vi "Scale_FPGA_Output_To_Volts.vi"(7 "Chan#":T8, 10 "FPGA_Data":ext[](array[numeric]), 11 "FP_User":T1={"#NoiseSums"=0, "Max_df"=0, "AvgAvg"=FALSE, "#Avg"=0, "AutoCenter"=FALSE, "Inclin"={"Vmin"=0.0, "Vmax"=0.0, "Angle_min"=0.0, "Angle_max"=0.0, "Offset"=0.0, "Pos_Neg"=FALSE}, "1"={"Cal_"={"Fine"=0.0, "Coarse_"=0.0}, "Beac"={"Fine"=0.0, "Coarse_"=0.0}, "Scale"={"Step4"=0.0, "Step5"=0.0, "Step6"=0.0, "Step7"=0.0}, "Offset"=0.0, "Scale_Noise"=0.0, "Scale_Step1"=0.0, "Scale_In_RT"=0.0, "ScaleMeas"=0.0, "FreqsToRemove"=[], "Width"=[0, 1633], "ScaleMeasEnum"=enum."1", "FilterEnab"=enum."None"}, "2"={"Cal_"={"Fine"=0.0, "Coarse_"=0.0}, "Beac"={"Fine"=0.0, "Coarse_"=0.0}, "Scale"={"Step4"=0.0, "Step5"=0.0, "Step6"=0.0, "Step7"=0.0}, "Offset"=0.0, "Scale_Noise"=0.0, "Scale_Step1"=0.0, "Scale_In_RT"=0.0, "ScaleMeas"=0.0, "FreqsToRemove"=[], "Width"=[0, 1633], "ScaleMeasEnum"=enum."1", "FilterEnab"=enum."None"}, "3"={"Cal_"={"Fine"=0.0, "Coarse_"=0.0}, "Beac"={"Fine"=0.0, "Coarse_"=0.0}, "Scale"={"Step4"=0.0, "Step5"=0.0, "Step6"=0.0, "Step7"=0.0}, "Offset"=0.0, "Scale_Noise"=0.0, "Scale_Step1"=0.0, "Scale_In_RT"=0.0, "ScaleMeas"=0.0, "FreqsToRemove"=[], "Width"=[0, 1633], "ScaleMeasEnum"=enum."1", "FilterEnab"=enum."None"}, "4"={"Cal_"={"Fine"=0.0, "Coarse_"=0.0}, "Beac"={"Fine"=0.0, "Coarse_"=0.0}, "Scale"={"Step4"=0.0, "Step5"=0.0, "Step6"=0.0, "Step7"=0.0}, "Offset"=0.0, "Scale_Noise"=0.0, "Scale_Step1"=0.0, "Scale_In_RT"=0.0, "ScaleMeas"=0.0, "FreqsToRemove"=[], "Width"=[0, 1633], "ScaleMeasEnum"=enum."1", "FilterEnab"=enum."None"}, "Target to Probe"=enum."1", "SNR_Thresh"=0.0, "Paths"={"CfgFile"=path "", "LogFolder"=path "", "LogFile"=path "", "NAS path"=path "", "ThreshFile"=path "", "RedunFolder"=path ""}, "Connex_Location"="", "SimulateFPGA"=FALSE, "Deadband"=0.0} {"Deadband" format="%#.0f"}) -> (2 "VoltsScalar":dbl, 3 "Time Domain Volts":ext[](array[numeric]))   [LabVIEW 2018]
uses:
  Controls/Enums/TargetNumber.ctl
  Controls/Clusts/FrontPanel_UserConfig.ctl
  Controls/Clusts/Inclinometer_User_Cfg.ctl
  Controls/Clusts/FP_UserTargetConfig.ctl
  Controls/Clusts/FreqShift.ctl
  Controls/Clusts/FPGA_Scale.ctl
  Controls/Enums/ScaleMeasure.ctl
  Controls/RadioButtons/FilterEnableRadio.ctl
  Controls/PathsCluster.ctl
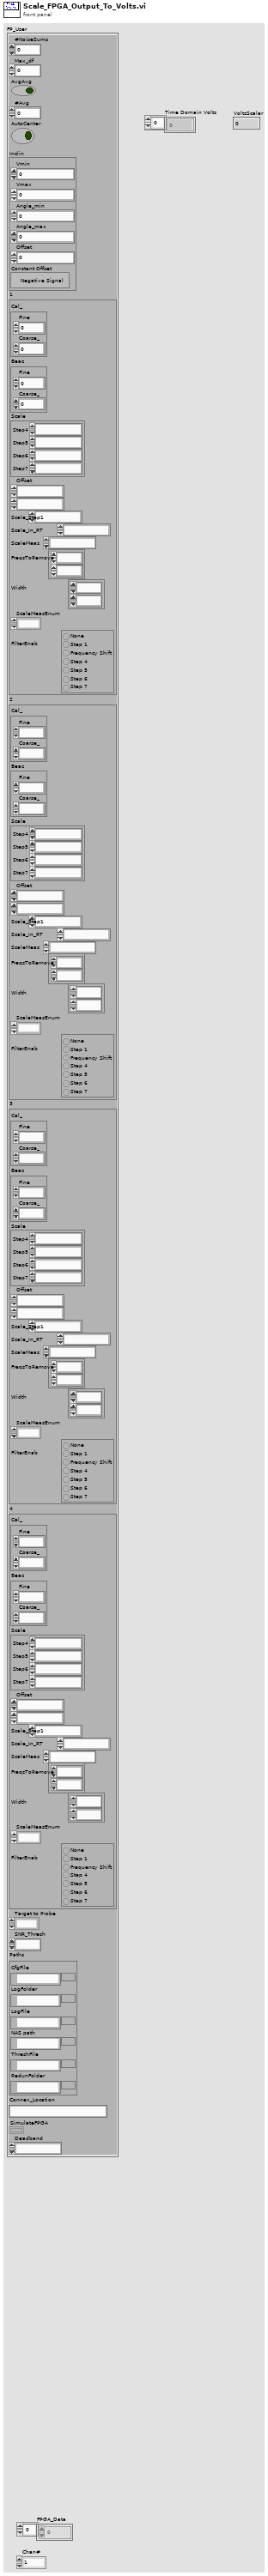
[diagram p1: front panel]
types:
  T1 = typedef "FrontPanel_UserConfig.ctl" = cluster{"#NoiseSums":u32, "Max_df":u32, "AvgAvg":bool, "#Avg":u16, "AutoCenter":bool, "Inclin":T2, "1":T3, "2":T3, "3":T3, "4":T3, "Target to Probe":T8, "SNR_Thresh":dbl, "Paths":T9, "Connex_Location":string, "SimulateFPGA":bool, "Deadband":dbl}
  T2 = typedef "Inclinometer_User_Cfg.ctl" = cluster{"Vmin":dbl, "Vmax":dbl, "Angle_min":dbl, "Angle_max":dbl, "Offset":dbl, "Pos_Neg":bool}
  T3 = typedef "FP_UserTargetConfig.ctl" = cluster{"Cal_":T4, "Beac":T4, "Scale":T5, "Offset":fxp<+/-,16,16>, "Scale_Noise":fxp<+/-,30,30>, "Scale_Step1":fxp<+/-,17,17>, "Scale_In_RT":ext, "ScaleMeas":fxp<+/-,16,1>, "FreqsToRemove":i32[], "Width":i32[], "ScaleMeasEnum":T6, "FilterEnab":T7}
  T4 = typedef "FreqShift.ctl" = cluster{"Fine":dbl, "Coarse_":dbl}
  T5 = typedef "FPGA_Scale.ctl" = cluster{"Step4":fxp<+/-,23,23>, "Step5":fxp<+/-,23,23>, "Step6":fxp<+/-,23,23>, "Step7":fxp<+/-,23,23>}
  T6 = typedef "ScaleMeasure.ctl" = enum16{"1", "10", "50", "42"}
  T7 = typedef "FilterEnableRadio.ctl" = enum32{"None", "Step 1", "Frequency Shift", "Step 4", "Step 5", "Step 6", "Step 7"}
  T8 = typedef "TargetNumber.ctl" = enum16{"1", "2", "3", "4"}
  T9 = typedef "PathsCluster.ctl" = cluster{"CfgFile":path, "LogFolder":path, "LogFile":path, "NAS path":path, "ThreshFile":path, "RedunFolder":path}
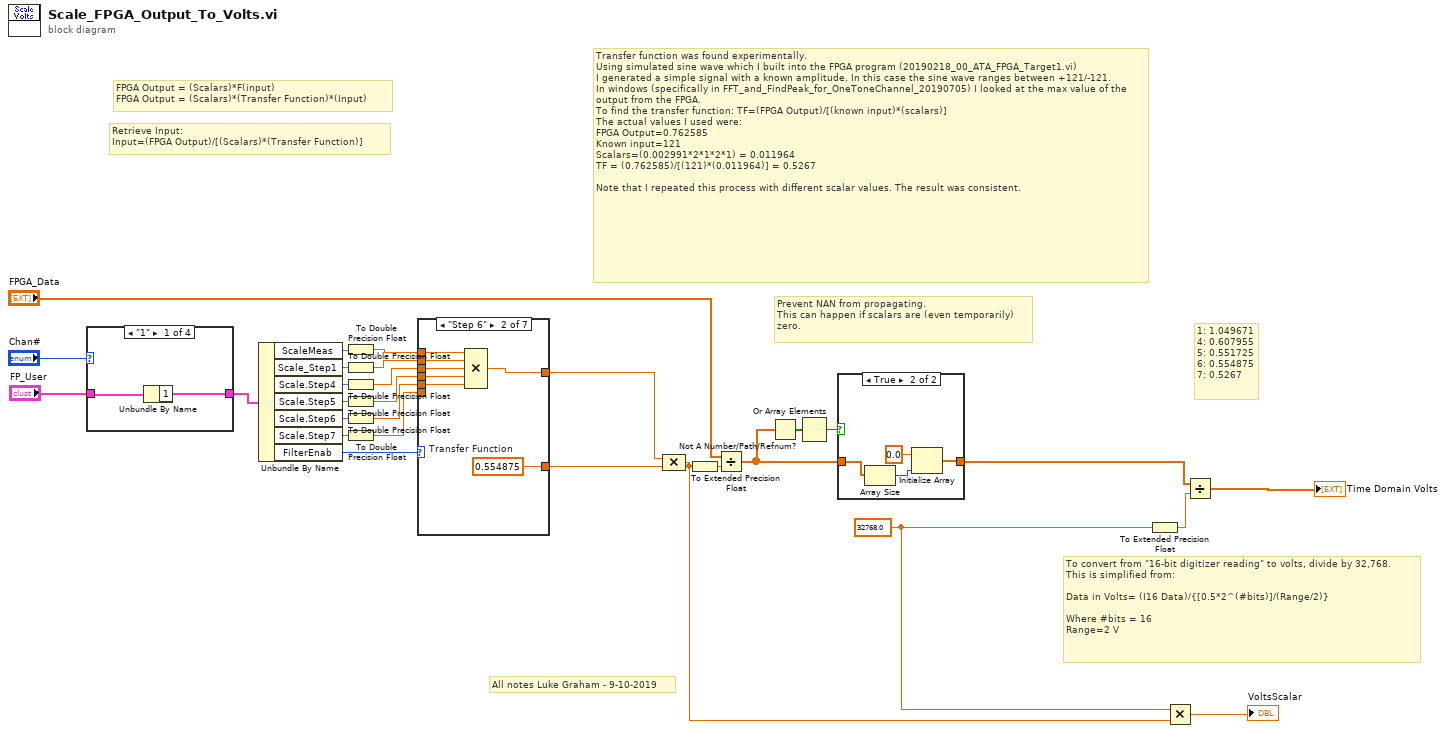
[diagram p0: block diagram]
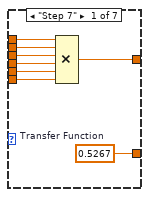
[diagram p3: hidden frame]
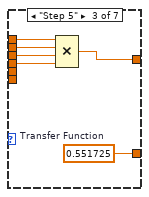
[diagram p4: hidden frame]
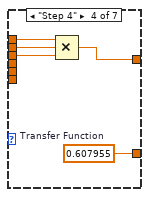
[diagram p5: hidden frame]
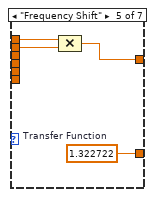
[diagram p6: hidden frame]
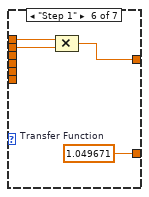
[diagram p7: hidden frame]
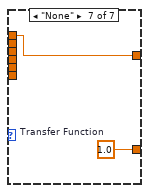
[diagram p8: hidden frame]
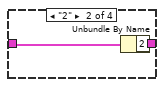
[diagram p9: hidden frame]
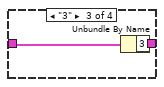
[diagram p10: hidden frame]
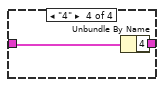
[diagram p11: hidden frame]
diagram:
  w8 = 32768.0 ("value")
  # "Prevent NAN from propagating.\nThis can happen if scalars are (even temporarily)\nzero."
  # "1: 1.049671\n4: 0.607955\n5: 0.551725\n6: 0.554875 \n7: 0.5267"
  # "All notes Luke Graham - 9-10-2019"
  # "To convert from \"16-bit digitizer reading\" to volts, divide by 32,768.\nThis is simplified from:\n\nData in Volts= (I16 Data)/{[0.5*2^(#bits)]/(Range/2)}\n\nWhere #bits = 16\nRange=2 V"
  # "Transfer function was found experimentally.\nUsing simulated sine wave which I built into the FPGA program (20190218_00_ATA_FPGA_Target1.vi)\nI generated a simple signal with a known amplitude. In this case the sine wave ranges between +121/-121.\nIn windows (specifically in FFT_and_FindPeak_for_OneToneChannel_20190705) I looked at the max value of the output from the FPGA. \nTo find the transfer function: TF=(FPGA Output)/[(known input)*(scalars)]\nThe actual values I used were:\nFPGA Output=0.762585\nKnown input=121\nScalars=(0.002991*2*1*2*1) = 0.011964\nTF = (0.762585)/[(121)*(0.011964)] = 0.5267\n\nNote that I repeated this process with different scalar values. The result was consistent."
  # "Retrieve Input:\nInput=(FPGA Output)/[(Scalars)*(Transfer Function)]"
  # "FPGA Output = (Scalars)*F(input)\nFPGA Output = (Scalars)*(Transfer Function)*(Input)"
  n1 = case shown="\"1\"" "Chan#" {
    tunnel: "FP_User" -> [w31 w33 w35 w37]
    tunnel: [w30 w32 w34 w36] -> w12
    frame "1" {
      n2 = Unbundle By Name(w31) -> ("1"=w30:T3)
    }
    frame "2" {
      n3 = Unbundle By Name(w33) -> ("2"=w32:T3)
    }
    frame "3" {
      n4 = Unbundle By Name(w35) -> ("3"=w34:T3)
    }
    frame "4" {
      n5 = Unbundle By Name(w37) -> ("4"=w36:T3)
    }
  }
  n6 = Unbundle By Name(w12) -> ("ScaleMeas"=w13:fxp<+/-,16,1>, "Scale_Step1"=w14:fxp<+/-,17,17>, "Scale.Step4"=w15:fxp<+/-,23,23>, "Scale.Step5"=w16:fxp<+/-,23,23>, "Scale.Step6"=w17:fxp<+/-,23,23>, "Scale.Step7"=w18:fxp<+/-,23,23>, "FilterEnab"=w5:T7)
  n7 = To Double Precision Float(number=w13) -> (double precision float=w19:dbl)
  n8 = To Double Precision Float(number=w14) -> (double precision float=w20:dbl)
  n9 = To Double Precision Float(number=w15) -> (double precision float=w21:dbl)
  n10 = To Double Precision Float(number=w16) -> (double precision float=w22:dbl)
  n11 = To Double Precision Float(number=w17) -> (double precision float=w23:dbl)
  n12 = To Double Precision Float(number=w18) -> (double precision float=w24:dbl)
  n13 = case shown="\"Step 6\"" w5 {
    tunnel: [w45 w52 w58 w63 w67 w71 w73] -> w26
    tunnel: [w44 w51 w57 w62 w66 w70 w72] -> w25
    tunnel: w24 -> [w43 _ _ _ _ _ _]
    tunnel: w23 -> [w42 w50 _ _ _ _ _]
    tunnel: w22 -> [w41 w49 w56 _ _ _ _]
    tunnel: w21 -> [w40 w48 w55 w61 _ _ _]
    tunnel: w20 -> [w39 w47 w54 w60 w65 w69 _]
    tunnel: w19 -> [w38 w46 w53 w59 w64 w68 w72]
    frame "Step 7" {
      w45 = 0.5267  # Transfer Function
      n14 = Compound Arithmetic op=MULTIPLY(w38, w39, w40, w41, w42, w43) -> (w44:dbl)
    }
    frame "Step 6" {
      w52 = 0.554875  # Transfer Function
      n15 = Compound Arithmetic op=MULTIPLY(w46, w47, w48, w49, w50) -> (w51:dbl)
    }
    frame "Step 5" {
      w58 = 0.551725  # Transfer Function
      n16 = Compound Arithmetic op=MULTIPLY(w53, w54, w55, w56) -> (w57:dbl)
    }
    frame "Step 4" {
      w63 = 0.607955  # Transfer Function
      n17 = Compound Arithmetic op=MULTIPLY(w59, w60, w61) -> (w62:dbl)
    }
    frame "Frequency Shift" {
      w67 = 1.322722  # Transfer Function
      n18 = Compound Arithmetic op=MULTIPLY(w64, w65) -> (w66:dbl)
    }
    frame "Step 1" {
      w71 = 1.049671  # Transfer Function
      n19 = Compound Arithmetic op=MULTIPLY(w68, w69) -> (w70:dbl)
    }
    frame "None" {
      w73 = 1.0  # Transfer Function
    }
  }
  n20 = Compound Arithmetic op=MULTIPLY(w25, w26) -> (w9:dbl)
  n21 = To Extended Precision Float(1:w9) -> (0:w28:ext)
  n22 = Divide(x="FPGA_Data", y=w28) -> (x/y=w3:ext[])
  n23 = Not A Number/Path/Refnum?(number/path/refnum=w3) -> (NaN/Path/Refnum?=w4:bool[])
  n24 = Or Array Elements(Boolean array=w4) -> (logical OR=w2:bool)
  n25 = case shown="True" w2 {
    tunnel: w3 -> [w74 w78]
    tunnel: [w74 w76] -> w1
    frame False {
    }
    frame True {
      n26 = Array Size(array=w78) -> (size(s)=w77:i32)
      n27 = Initialize Array(0.0 ("element"), w77) -> (w76:dbl[])
    }
  }
  n28 = To Extended Precision Float(1:w8) -> (0:w7:ext)
  n29 = Multiply(x=w8, y=w9) -> (x*y=→"VoltsScalar":dbl)
  n30 = Divide(x=w1, y=w7) -> (x/y=→"Time Domain Volts":ext[])
